vi "Read Cell Housekeeping Data.vi"(8 "error in":errorcluster, 11 "PAS Data in":refnum<class "PAS Data.lvclass">=refnum) -> (0 "error out":errorcluster, 2 "houseKeeping":T1, 3 "PAS Data out":refnum<class "PAS Data.lvclass">)   [LabVIEW 2014, in "PAS Data.lvclass"]
uses:
  PAS Data.lvclass
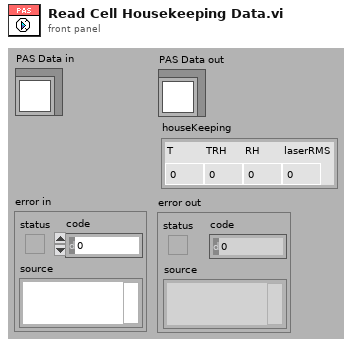
[diagram p1: front panel]
types:
  T1 = cluster{"T":sgl, "TRH":sgl, "RH":sgl, "laserRMS":sgl}
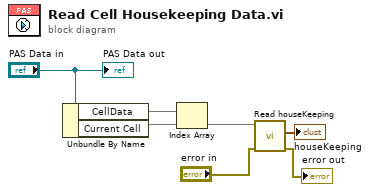
[diagram p0: block diagram]
diagram:
  n1 = Unbundle By Name("PAS Data in") -> ("CellData"=w5, "Current Cell"=w6)
  n2 = Index Array(array=w5, index=w6) -> (element=w4)
  n3 = call "Read houseKeeping.vi"("error in (no error)"="error in", "PAS Cell Data in"=w4) -> ("error out"=→"error out":errorcluster, "houseKeeping"=→"houseKeeping":T1)  [unwired: 7 in, 1 out]
  "PAS Data out" <- "PAS Data in"
